vi "UpOpenNode.vi"(10 "node ref in":refnum<data-value>, 11 "RVCLibrary_Bug2 in":refnum<class "RVCLibrary_Bug2.lvclass">) -> (2 "node ref out":refnum<data-value>, 3 "RVCLibrary_Bug2 out":refnum<class "RVCLibrary_Bug2.lvclass">)   [LabVIEW 2013, in "RVCLibrary_Bug2.lvclass"]
uses:
  RVCLibrary_Bug2.lvclass
  <vilib>/robotics/Navigation/shared/MapNode/AbstractDstarNode/NI_Robotics_AbstractDstarNode.lvclass
  RVCLibrary_Bug2.lvclass/RVCLibrary_Bug2.ctl
  <vilib>/robotics/Navigation/shared/Priority Queue/NI_Robotics_Priority Queue.lvclass
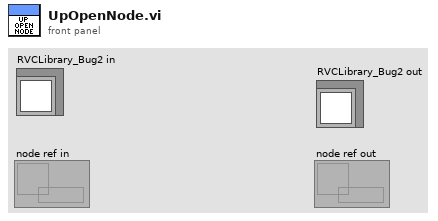
[diagram p1: front panel]
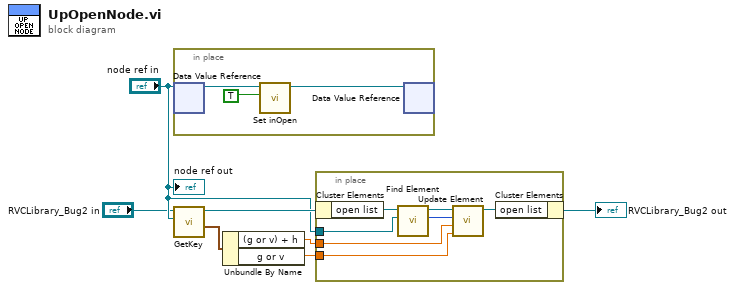
[diagram p0: block diagram]
diagram:
  n1 = in-place {
    n2 = in-place-dvr #1("node ref in") -> (w9:refnum<class "NI_Robotics_AbstractDstarNode.lvclass">)  [unwired: 1 out]
    n3 = call <vilib>:"Set inOpen.vi"("inOpen"=TRUE, "AbstractDstarNode in"=w9) -> ("AbstractDstarNode out"=w8:refnum<class "NI_Robotics_AbstractDstarNode.lvclass">)  [unwired: 8 in, 1 out]
    n4 = in-place-dvr #1(w8) -> ()  [unwired: 2 out]
  }
  n5 = call "GetKey.vi"("node ref in"="node ref in", "RVCLibrary_Bug2 in"="RVCLibrary_Bug2 in") -> ("key out"=w6:cluster{"(g or v) + h":dbl, "g or v":dbl}, "RVCLibrary_Bug2 out"=w7:refnum<class "RVCLibrary_Bug2.lvclass">)  [unwired: 7 in, 1 out]
  n6 = Unbundle By Name(w6) -> ("(g or v) + h"=w5:dbl, "g or v"=w4:dbl)
  n7 = in-place {
    in-place-border: "node ref in" -> [w17]
    in-place-border: w5 -> [w13]
    in-place-border: w4 -> [w12]
    n8 = in-place-cluster #2(w7) -> ("open list"=w16:refnum<class "NI_Robotics_Priority Queue.lvclass">)
    n9 = call <vilib>:"Find Element.vi"("node Ref"=w17, "Priority Queue in"=w16) -> ("Numeric"=w14:i32, "Priority Queue out"=w15:refnum<class "NI_Robotics_Priority Queue.lvclass">)  [unwired: 7 in, 1 out]
    n10 = call <vilib>:"Update Element.vi"("g"=w12, "f"=w13, "index"=w14, "Priority Queue in"=w15) -> ("Priority Queue out"=w11:refnum<class "NI_Robotics_Priority Queue.lvclass">)  [unwired: 7 in]
    n11 = in-place-cluster #2("open list"=w11) -> (→"RVCLibrary_Bug2 out":refnum<class "RVCLibrary_Bug2.lvclass">)
  }
  "node ref out" <- "node ref in"
